vi "Write Display Controls.vi"(8 "error in (no error)":errorcluster, 10 "Visible Controls":T1, 11 "teststand-api in":refnum<class "teststand-api.lvclass">) -> (0 "error out":errorcluster, 3 "teststand-api out":refnum<class "teststand-api.lvclass">)   [LabVIEW 2014, in "teststand-api.lvlib" / "teststand-api.lvclass"]
uses:
  teststand-api.lvclass
  TS Controls Argument--cluster.ctl
  teststand-api.lvclass/teststand-api.ctl
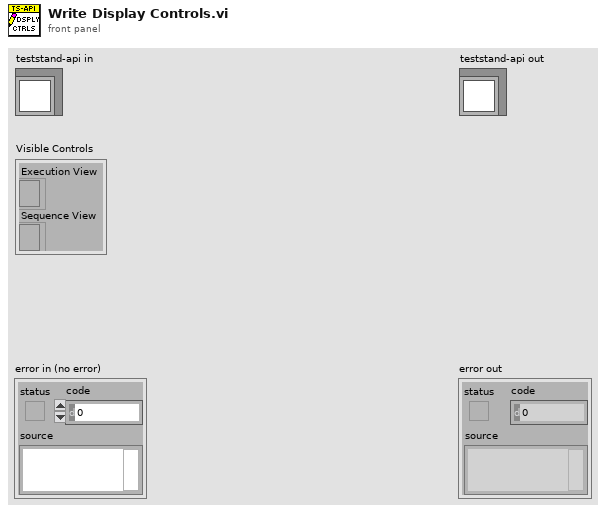
[diagram p1: front panel]
types:
  T1 = typedef "teststand-api.lvlib/teststand-api.lvclass/TS Controls Argument--cluster.ctl" = cluster{"Execution View":refnum<k7>, "Sequence View":refnum<k7>}
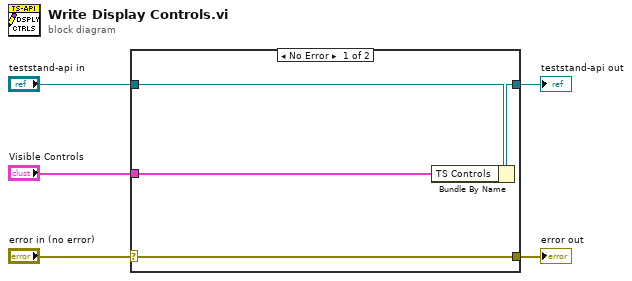
[diagram p0: block diagram]
diagram:
  n1 = case shown="No Error" "error in (no error)" {
    selector: "error in (no error)" -> [w9 w10]
    tunnel: [w9 w10] -> w4
    tunnel: [w7 w11] -> w2
    tunnel: "teststand-api in" -> [w8 w11]
    tunnel: "Visible Controls" -> [w6 _]
    frame No Error {
      n2 = Bundle By Name(cluster=w8, "TS Controls"=w6) -> (w7:refnum<class "teststand-api.lvclass">)
    }
    frame Error {
    }
  }
  "error out" <- w4
  "teststand-api out" <- w2
